vi "PDF Welding.vi"(0 "configuration file path":path caption="配置文件的路径", 1 "PDF Welding msic inf":T1) -> ()   [LabVIEW 2014]
uses:
  Ctl.xio/PDF Welding msic ctl.ctl
  SubVIS.xio/DataSocket/DataSocket_Tags.ctl
  Ctl.xio/part type.ctl
  SubVIS.xio/DataSocket/Write PLC Vars/Write Bool Var in.vi
  <vilib>/Utility/file.llb/Read From Spreadsheet File (string).vi
  SubVIS.xio/DataSocket/Write PLC Vars/Write String Var in.vi
  SubVIS.xio/DataSocket/Read PLC Vars/Read Bool Var.vi
  SubVIS.xio/DataSocket/Read PLC Vars/Read U32 Var.vi
  SubVIS.xio/DataSocket/Write PLC Vars/Write Dbl Var in.vi
  SubVIS.xio/Hopper car inf/Curing inf.vi
panel:
  in  "SQL information":string
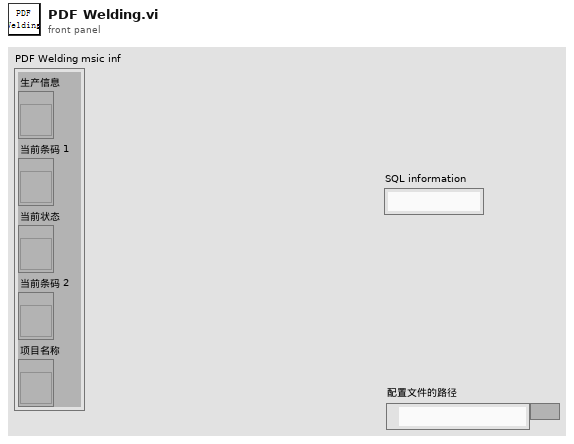
[diagram p1: front panel]
types:
  T1 = cluster{"生产信息":refnum<vi>, "当前条码 1":refnum<vi>, "当前状态":refnum<vi>, "当前条码 2":refnum<vi>, "项目名称":refnum<vi>}
  T2 = typedef "PDF Welding msic ctl.ctl" = cluster{"configuration file path":path, "DsOut":T3[], "Hopper car information":cluster{"Hopper car code":string, "Hopper car No":string, "plate No":string}, "pallet.produced number":i32, "SQL information":string, "Serial number":i32, "database path":path, "PDF Welding msic inf":cluster{"生产信息":refnum<vi>, "当前条码 1":refnum<vi>, "当前状态":refnum<vi>, "当前条码 2":refnum<vi>, "项目名称":refnum<vi>}, "Heating process parameters":cluster{"heating start":string, "heating finish":string, "Heating time use":u32}, "part type":T4, "Inlet temperature database":string[], "Outlet temperature database":string[], "Inlet temperature buffer":i32[], "Outlet temperature buffer":i32[], "PDF start time":string, "PDF finish time":string, "BarCode1":string, "BarCode2":string, "scanner resource name out":refnum<visa-resource-name>, "scanner coms or ip":string, "Outlet pressure buffer":i32[], "Outlet pressure database":string[], "scanner ip ID":refnum<k5>}
  T3 = typedef "DataSocket_Tags.ctl" = cluster{"Ds ID":refnum<k13>, "Tag":string}
  T4 = typedef "part type.ctl" = cluster{"项目号":string, "物料代码":string, "零件号":string, "供应商编码":string, "产线编码":string, "客户代码":string, "颜色代码":string, "托盘上限":i32, "加热温度":string, "加热时长":string, "EOL Stations":string}
  T5 = cluster{"Hopper car code":string, "Hopper car No":string, "plate No":string}
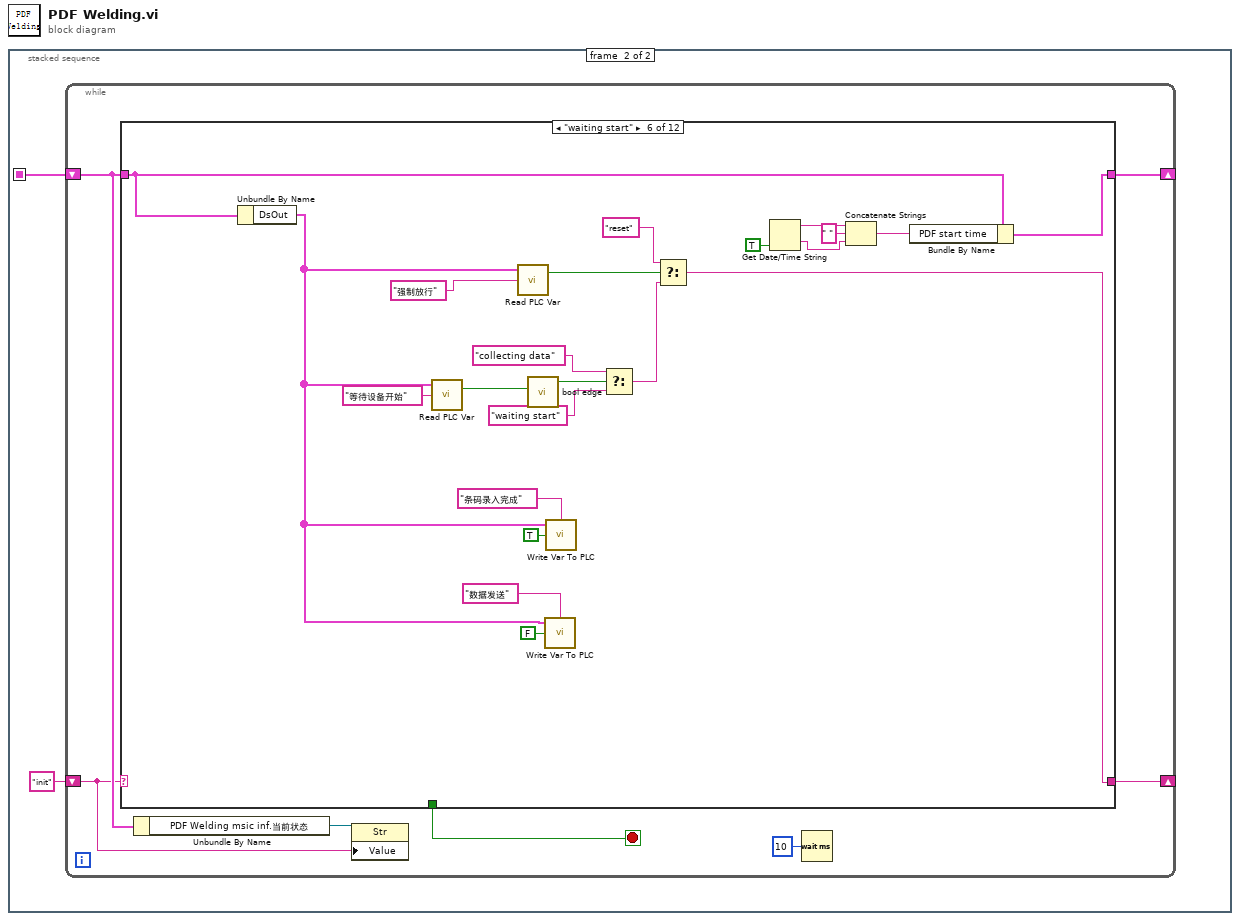
[diagram p0: block diagram]
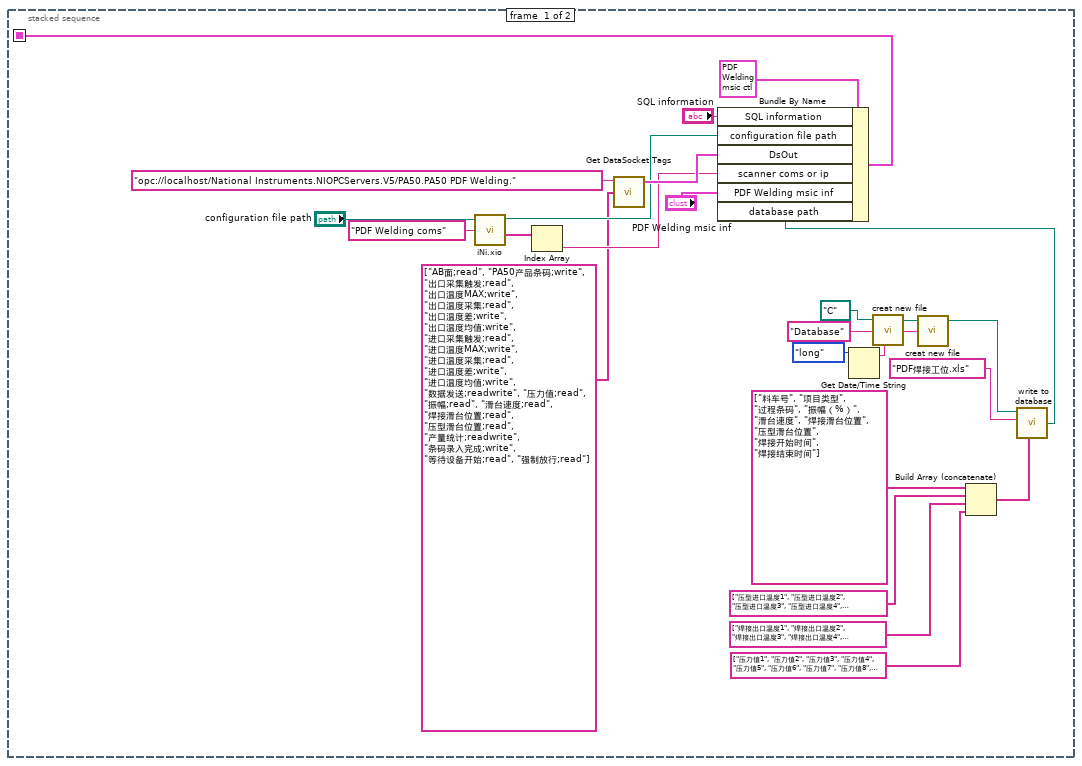
[diagram p2: hidden frame]
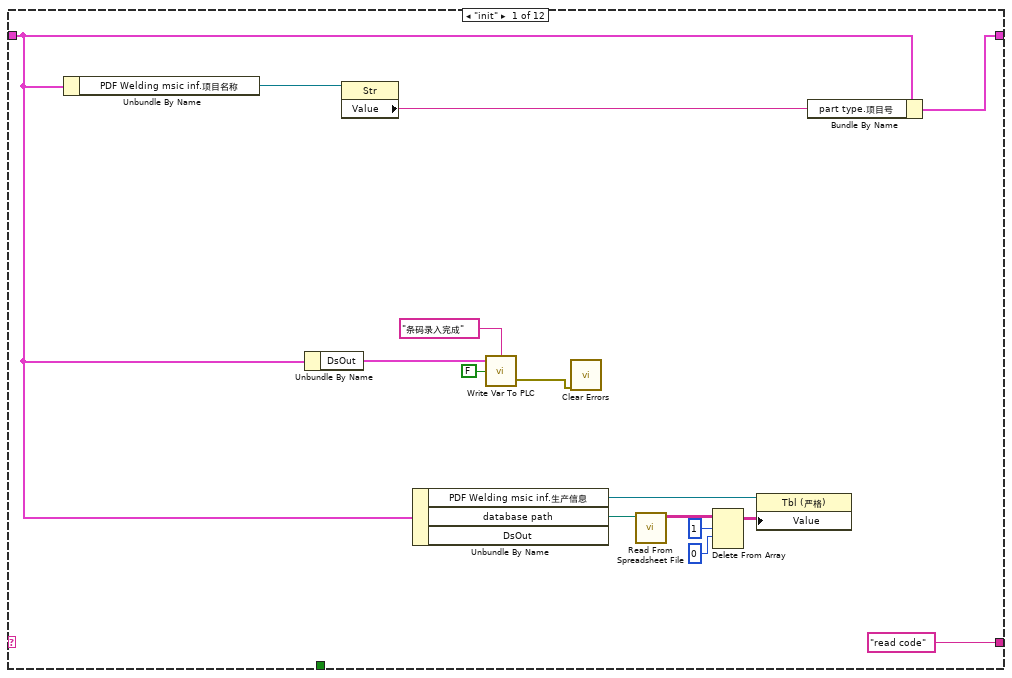
[diagram p3: hidden frame]
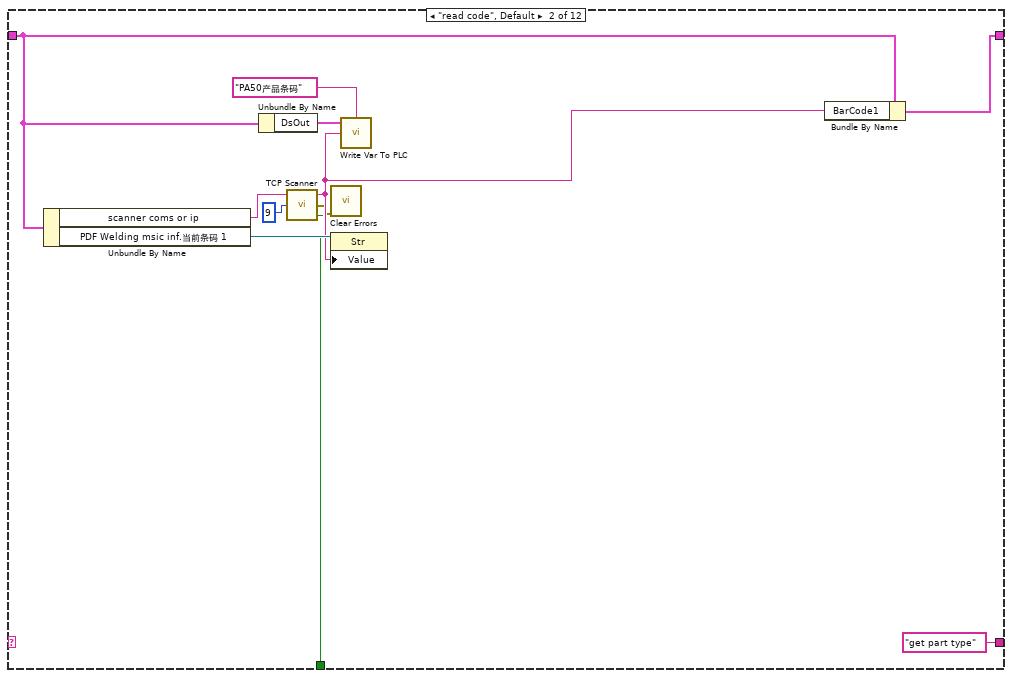
[diagram p4: hidden frame]
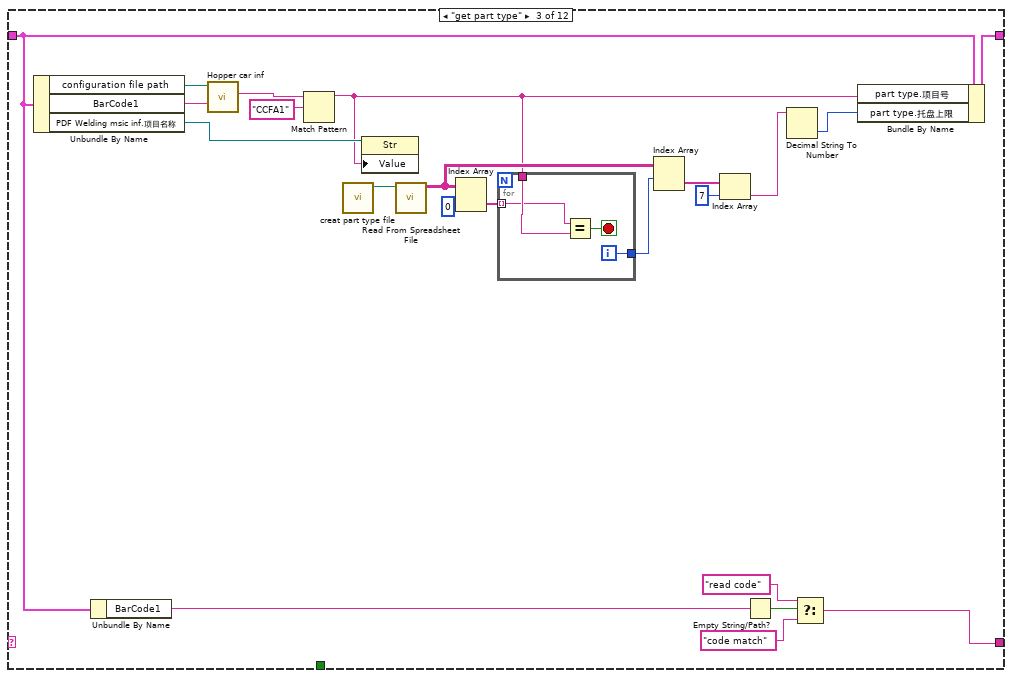
[diagram p5: hidden frame]
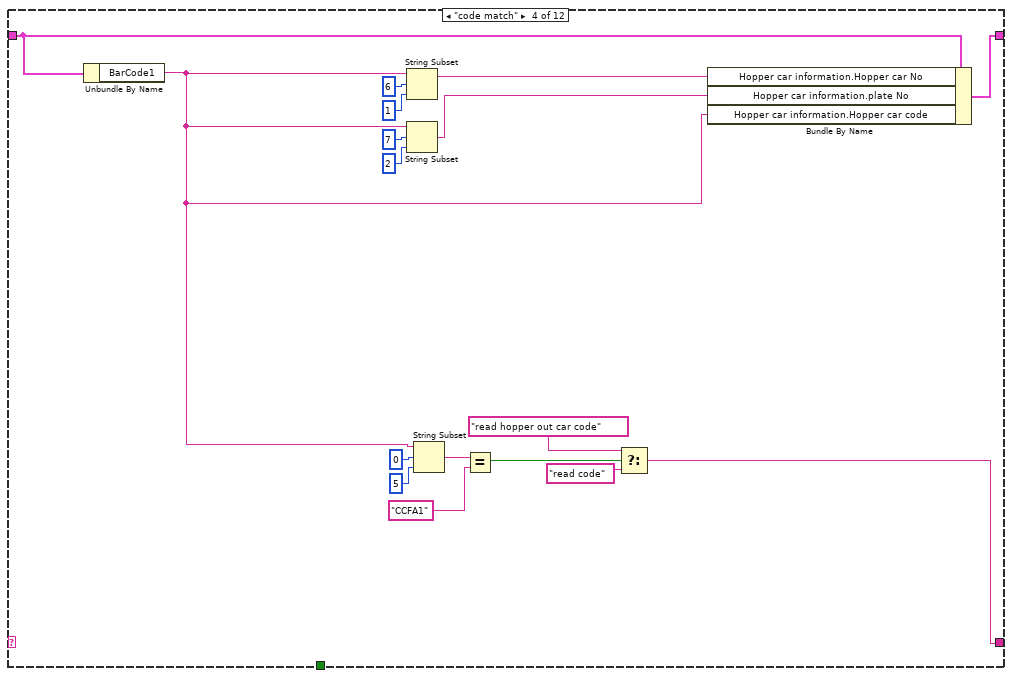
[diagram p6: hidden frame]
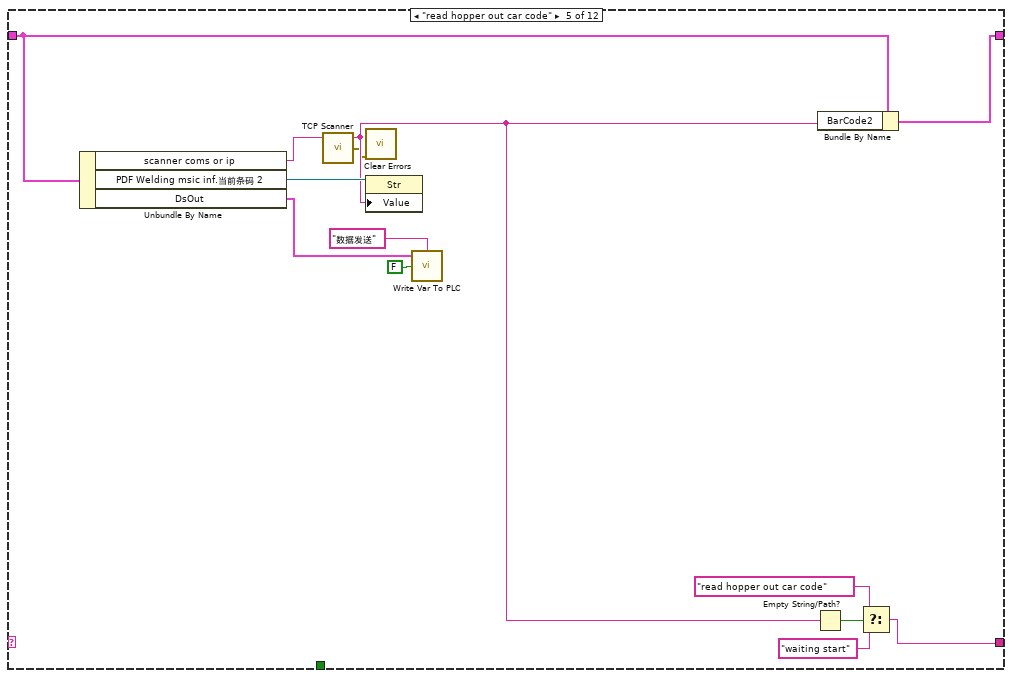
[diagram p7: hidden frame]
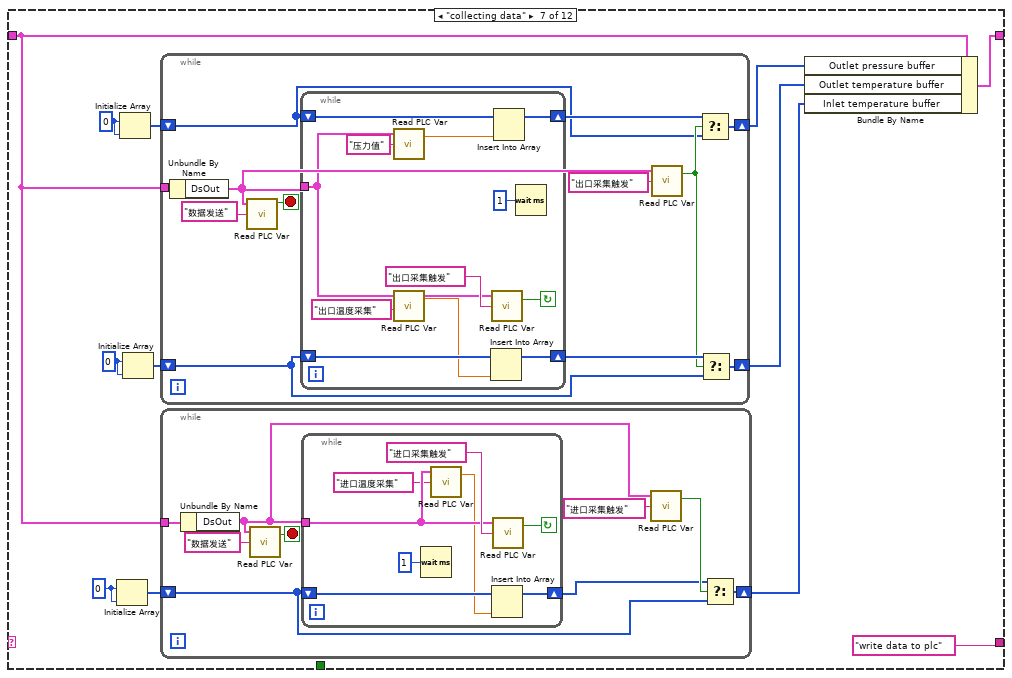
[diagram p8: hidden frame]
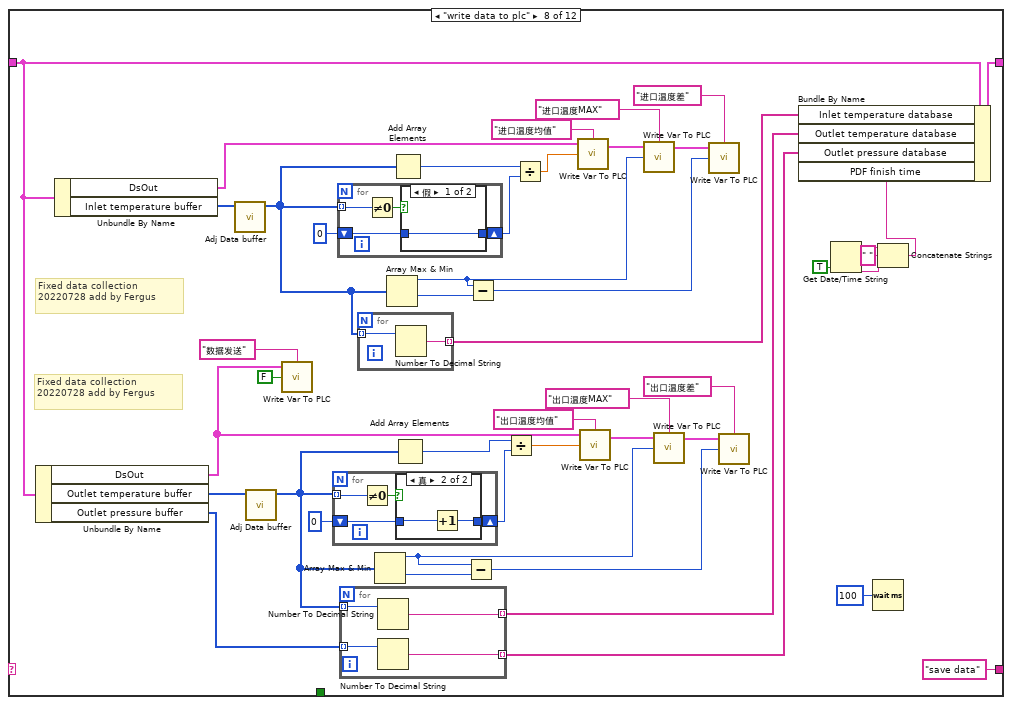
[diagram p9: hidden frame]
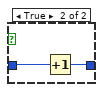
[diagram p11: hidden frame]
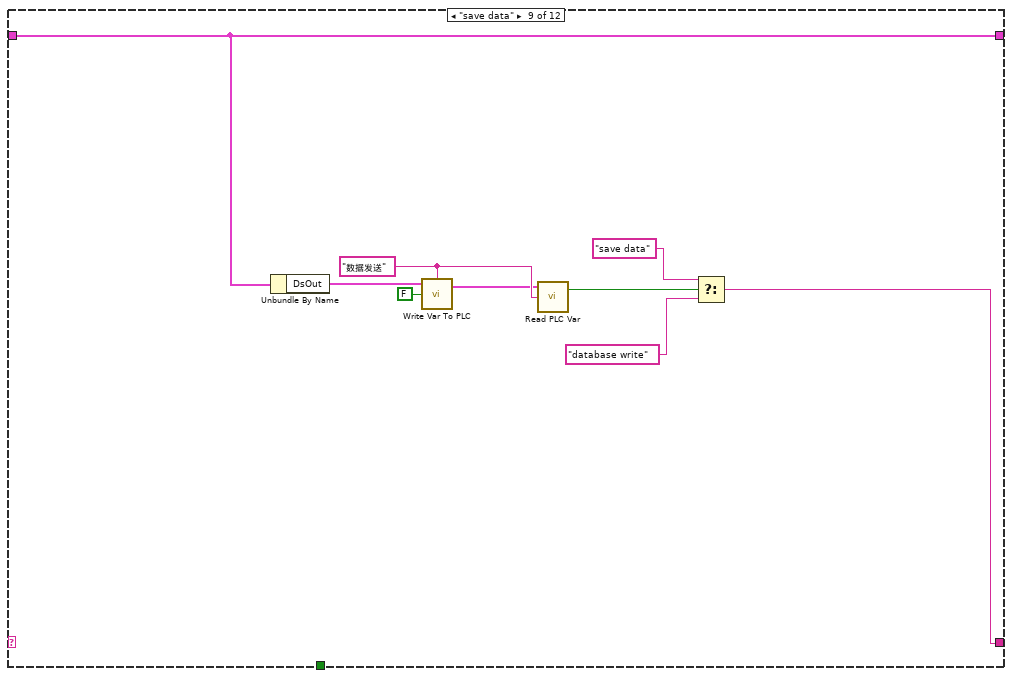
[diagram p12: hidden frame]
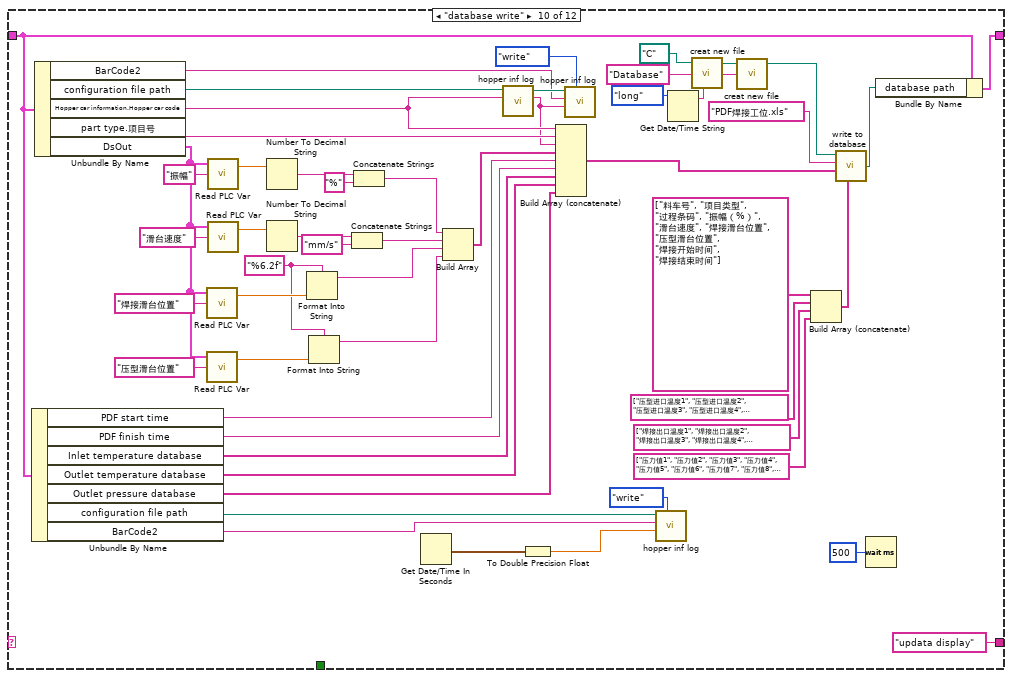
[diagram p13: hidden frame]
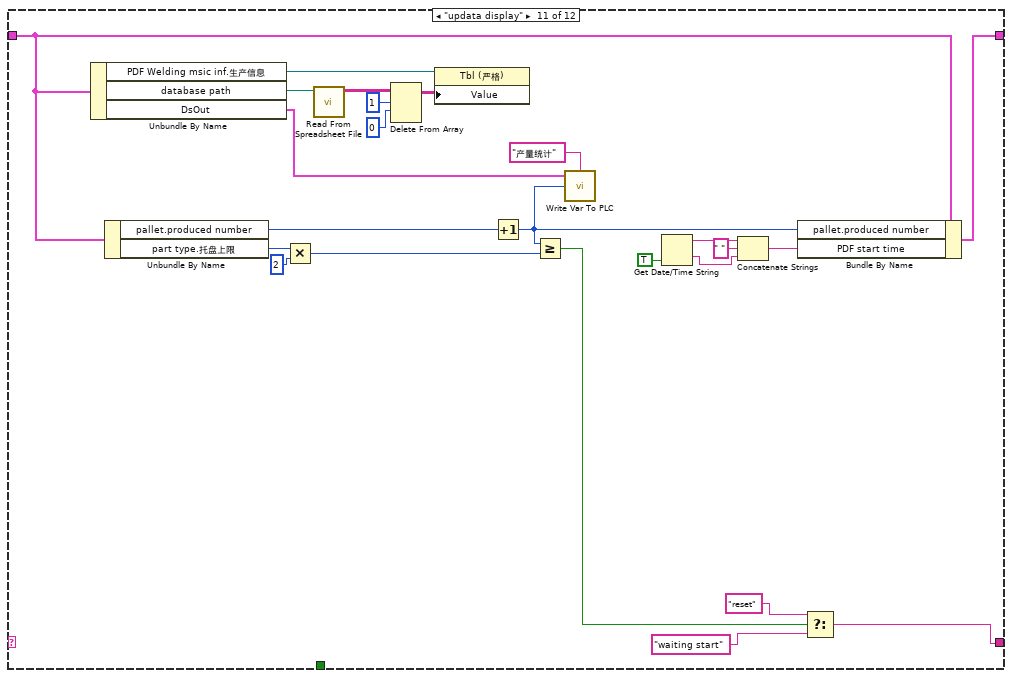
[diagram p14: hidden frame]
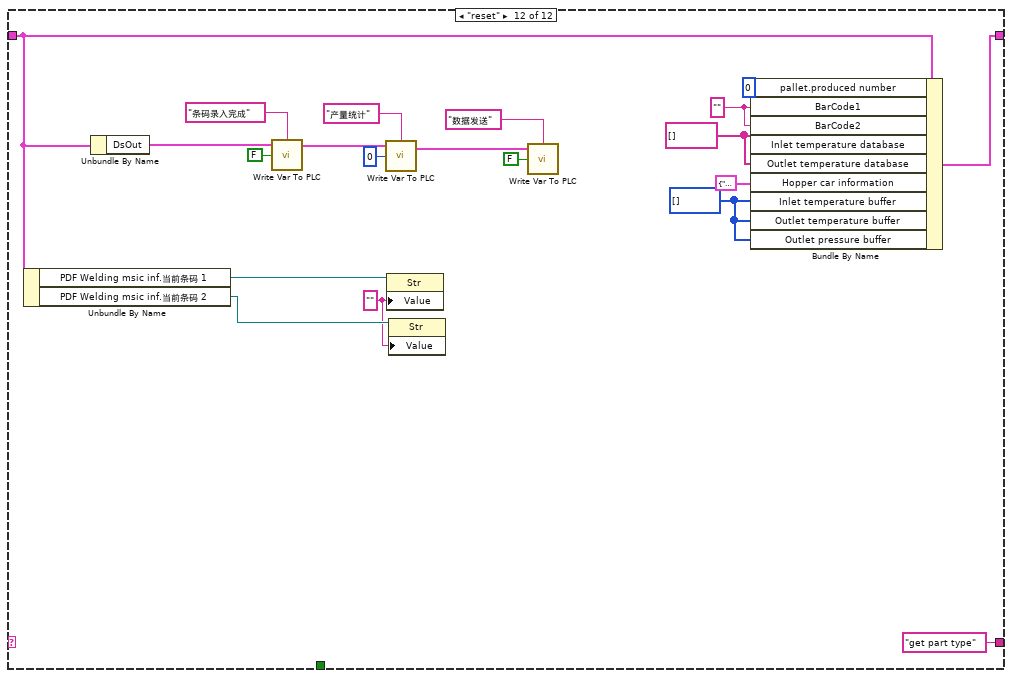
[diagram p15: hidden frame]
diagram:
  n1 = stacked-sequence {
    seq-local: [w14 _] -> [_ w26]
    frame #0 {
      n2 = call "iNi.xio.vi"("configuration file path"="configuration file path", "Sections"="PDF Welding coms") -> ("configuration file path"=w24:path, "Values"=w22:string[])  [unwired: 1 in, 3 out]
      n3 = Index Array(array=w22) -> (element=w21:string)  [unwired: 1 in]
      n4 = call "Get DataSocket Tags.vi"("All Tags"=string[] ["AB面;read", "PA50产品条码;write", "出口采集触发;read", "出口温度MAX;write", "出口温度采集;read", "出口温度差;write", "出口温度均值;write", "进口采集触发;read", "进口温度MAX;write", "进口温度采集;read", "进口温度差;write", "进口温度均值;write", "数据发送;readwrite", "压力值;read", "振幅;read", "滑台速度;read", "焊接滑台位置;read", "压型滑台位置;read", "产量统计;readwrite", "条码录入完成;write", "等待设备开始;read", "强制放行;read"], "URL"="opc://localhost/National Instruments.NIOPCServers.V5/PA50.PA50 PDF Welding.") -> ("DsOut"=w25:T3[])  [unwired: 3 in]
      n5 = Get Date/Time String(date format (0)=enum16{"short", "long", "abbreviated"}."long" ("日期格式(0)")) -> (date string=w8:string)  [unwired: 2 in, 1 out]
      n6 = call "creat new file.vi"("file name"="Database", "path"=path "C:/") -> ("created path"=w10:path)  [unwired: 1 in, 2 out]
      n7 = call "creat new file.vi"("file name"=w8, "path"=w10) -> ("created path"=w9:path)  [unwired: 1 in, 2 out]
      n8 = Build Array (concatenate)(string[] ["料车号", "项目类型", "过程条码", "振幅（%）", "滑台速度", "焊接滑台位置", "压型滑台位置", "焊接开始时间", "焊接结束时间"] ("Header"), string[] ["压型进口温度1", "压型进口温度2", "压型进口温度3", "压型进口温度4", "压型进口温度5", "压型进口温度6", "压型进口温度7", "压型进口温度8", "压型进口温度9", "压型进口温度10", "压型进口温度11", "压型进口温度12", "压型进口温度13", "压型进口温度14", "压型进口温度15", "压型进口温度16", "压型进口温度17", "压型进口温度18", "压型进口温度19", "压型进口温度20", "压型进口温度21", "压型进口温度22", "压型进口温度23", "压型进口温度24", "压型进口温度25", "压型进口温度26", "压型进口温度27", "压型进口温度28", "压型进口温度29", "压型进口温度30"] ("数组"), string[] ["焊接出口温度1", "焊接出口温度2", "焊接出口温度3", "焊接出口温度4", "焊接出口温度5", "焊接出口温度6", "焊接出口温度7", "焊接出口温度8", "焊接出口温度9", "焊接出口温度10", "焊接出口温度11", "焊接出口温度12", "焊接出口温度13", "焊接出口温度14", "焊接出口温度15", "焊接出口温度16", "焊接出口温度17", "焊接出口温度18", "焊接出口温度19", "焊接出口温度20", "焊接出口温度21", "焊接出口温度22", "焊接出口温度23", "焊接出口温度24", "焊接出口温度25", "焊接出口温度26", "焊接出口温度27", "焊接出口温度28", "焊接出口温度29", "焊接出口温度30"] ("数组"), string[] ["压力值1", "压力值2", "压力值3", "压力值4", "压力值5", "压力值6", "压力值7", "压力值8", "压力值9", "压力值10", "压力值11", "压力值12", "压力值13", "压力值14", "压力值15", "压力值16", "压力值17", "压力值18", "压力值19", "压力值20", "压力值21", "压力值22", "压力值23", "压力值24", "压力值25", "压力值26", "压力值27", "压力值28", "压力值29", "压力值30"] ("数组 2")) -> (w6:string[])
      n9 = call "write to database.vi"("Header"=w6, "file name"="PDF焊接工位.xls", "path"=w9) -> ("new file path (Not A Path if cancelled)"=w3:path)  [unwired: 3 in]
      n10 = Bundle By Name(cluster=T2 {"configuration file path"=path "", "DsOut"=[], "Hopper car information"={"Hopper car code"="", "Hopper car No"="", "plate No"=""}, "pallet.produced number"=0, "SQL information"="", "Serial number"=0, "database path"=path "", "PDF Welding msic inf"={"生产信息"=refnum, "当前条码 1"=refnum, "当前状态"=refnum, "当前条码 2"=refnum, "项目名称"=refnum}, "Heating process parameters"={"heating start"="", "heating finish"="", "Heating time use"=0}, "part type"={"项目号"="", "物料代码"="", "零件号"="", "供应商编码"="", "产线编码"="", "客户代码"="", "颜色代码"="", "托盘上限"=0, "加热温度"="", "加热时长"="", "EOL Stations"=""}, "Inlet temperature database"=[], "Outlet temperature database"=[], "Inlet temperature buffer"=[], "Outlet temperature buffer"=[], "PDF start time"="", "PDF finish time"="", "BarCode1"="", "BarCode2"="", "scanner resource name out"="", "scanner coms or ip"="", "Outlet pressure buffer"=[], "Outlet pressure database"=[], "scanner ip ID"=refnum} ("PDF Welding msic ctl"), "SQL information"="SQL information", "configuration file path"=w24, "DsOut"=w25, "scanner coms or ip"=w21, "PDF Welding msic inf"="PDF Welding msic inf", "database path"=w3) -> (w14:T2)
    }
    frame #1 {
      n11 = while {
        shift-right: [w34] -> _
        shift-left: w26 -> [w30]
        shift-right: [w33] -> _
        shift-left: "init" ("event") -> [w29]
        stop <- w28 stop-if-true
        n12 = case shown="\"waiting start\"" w29 {
          tunnel: w30 -> [w36 w57 w65 w89 w115 w119 w139 w207 w264 w308 w334 w353]
          tunnel: [w49 w60 w82 w97 w114 w117 w150 w208 w264 w314 w333 w362] -> w34
          tunnel: ["read code" "get part type" ("f") w69 w96 w108 w130 "write data to plc" ("f") "save data" ("f") w257 "updata display" ("f") w329 "get part type" ("f")] -> w33
          tunnel: [_ w50 _ _ _ _ _ _ _ _ _ _] -> w28
          frame "init" {
            n13 = Unbundle By Name(w36) -> ("PDF Welding msic inf.项目名称"=w48:refnum<vi>)
            n14 = Unbundle By Name(w36) -> ("DsOut"=w45:T3[])
            n15 = property class="Str"(reference=w48) -> ("Value"=w47:string)  [unwired: 1 in, 2 out]
            n16 = Unbundle By Name(w36) -> ("PDF Welding msic inf.生产信息"=w42:refnum<vi>, "database path"=w41:path)  [unwired: 1 out]
            n17 = call-poly "Write Var To PLC.vi"("Tag IN"="条码录入完成", "Bool Var in"=FALSE, "Ds PLCTags IN"=w45) -> ("error out"=w35:errorcluster)  [unwired: 1 in, 1 out]
            n18 = call <vilib>:"Clear Errors.vi"("error in (no error)"=w35) -> ()  [unwired: 5 in, 2 out]
            n19 = call-poly <vilib>:"Read From Spreadsheet File.vi"("file path (dialog if empty)"=w41) -> ("all rows"=w40:string[][])  [unwired: 6 in, 4 out]
            n20 = Delete From Array(array=w40, length=1 ("长度"), index (row)=0 ("索引 (行)")) -> (array with subset deleted=w37:string[][])  [unwired: 1 in, 1 out]
            n21 = property class="Tbl (严格)"(reference=w42, "Value"=w37) -> ()  [unwired: 1 in, 2 out]
            n22 = Bundle By Name(cluster=w36, "part type.项目号"=w47) -> (w49:T2)
          }
          frame "read code", Default {
            n23 = Unbundle By Name(w57) -> ("scanner coms or ip"=w53:string, "PDF Welding msic inf.当前条码 1"=w59:refnum<vi>)
            n24 = Unbundle By Name(w57) -> ("DsOut"=w56:T3[])
            n25 = call "TCP Scanner.vi"("byte of read(9)"=9 ("读取的字节"), "ip"=w53) -> ("status"=w50:bool, "错误输出"=w51:errorcluster, "Barcode"=w55:string)  [unwired: 1 in]
            n26 = call <vilib>:"Clear Errors.vi"("error in (no error)"=w51) -> ()  [unwired: 5 in, 2 out]
            n27 = property class="Str"(reference=w59, "Value"=w55) -> ()  [unwired: 1 in, 2 out]
            n28 = call-poly "Write Var To PLC.vi"("Tag IN"="PA50产品条码", "String Var in"=w55, "Ds PLCTags IN"=w56) -> ()  [unwired: 1 in, 2 out]
            n29 = Bundle By Name(cluster=w57, "BarCode1"=w55) -> (w60:T2)
          }
          frame "get part type" {
            n30 = Unbundle By Name(w65) -> ("configuration file path"=w67:path, "BarCode1"=w66:string, "PDF Welding msic inf.项目名称"=w64:refnum<vi>)
            n31 = Unbundle By Name(w65) -> ("BarCode1"=w68:string)
            n32 = call "Hopper car inf.vi"("key"=w66, "path in"=w67) -> ("value out"=w63:string)  [unwired: 8 in, 1 out]
            n33 = Match Pattern(string=w63, regular expression="CCFA1" ("正则表达式")) -> (before substring=w61:string)  [unwired: 1 in, 3 out]
            n34 = call "creat part type file.vi"() -> ("new file path (Not A Path if cancelled)"=w73:path)  [unwired: 11 in]
            n35 = property class="Str"(reference=w64, "Value"=w61) -> ()  [unwired: 1 in, 2 out]
            n36 = call-poly <vilib>:"Read From Spreadsheet File.vi"("file path (dialog if empty)"=w73) -> ("all rows"=w78:string[][])  [unwired: 6 in, 4 out]
            n37 = Index Array(array=w78, index (col)=0 ("禁用的索引 (列)")) -> (element=w80:string[])  [unwired: 1 in]
            n38 = for {
              tunnel: w80 -> [w83] mode=indexing
              tunnel: [w85] -> w77
              tunnel: w61 -> [w84]
              i -> [w85]
              stop <- w86 stop-if-true
              n39 = Equal?(x=w83, y=w84) -> (x = y?=w86:bool)
            }
            n40 = Index Array(array=w78, index (row)=w77) -> (element=w76:string[])  [unwired: 1 in]
            n41 = Index Array(array=w76, index=7 ("索引")) -> (element=w75:string)
            n42 = Empty String/Path?(string/path=w68) -> (empty?=w72:bool)
            n43 = Decimal String To Number(string=w75) -> (number=w74:i32)  [unwired: 2 in, 1 out]
            n44 = Select(t="read code", s=w72, f="code match") -> (s? t:f=w69:string)
            n45 = Bundle By Name(cluster=w65, "part type.项目号"=w61, "part type.托盘上限"=w74) -> (w82:T2)
          }
          frame "code match" {
            n46 = Unbundle By Name(w89) -> ("BarCode1"=w88:string)
            n47 = String Subset(string=w88, offset (0)=6 ("偏移量(0)"), length (rest)=1 ("长度（剩余）")) -> (substring=w91:string)
            n48 = String Subset(string=w88, offset (0)=7 ("偏移量(0)"), length (rest)=2 ("长度（剩余）")) -> (substring=w92:string)
            n49 = String Subset(string=w88, offset (0)=0 ("偏移量(0)"), length (rest)=5 ("长度（剩余）")) -> (substring=w93:string)
            n50 = Equal?(x=w93, y="CCFA1") -> (x = y?=w87:bool)
            n51 = Select(t="read hopper out car code" ("event"), s=w87, f="read code" ("event")) -> (s? t:f=w96:string)
            n52 = Bundle By Name(cluster=w89, "Hopper car information.Hopper car No"=w91, "Hopper car information.plate No"=w92, "Hopper car information.Hopper car code"=w88) -> (w97:T2)
          }
          frame "read hopper out car code" {
            n53 = Unbundle By Name(w115) -> ("scanner coms or ip"=w116:string, "PDF Welding msic inf.当前条码 2"=w113:refnum<vi>, "DsOut"=w104:T3[])
            n54 = call "TCP Scanner.vi"("ip"=w116) -> ("错误输出"=w107:errorcluster, "Barcode"=w109:string)  [unwired: 2 in, 1 out]
            n55 = call <vilib>:"Clear Errors.vi"("error in (no error)"=w107) -> ()  [unwired: 5 in, 2 out]
            n56 = property class="Str"(reference=w113, "Value"=w109) -> ()  [unwired: 1 in, 2 out]
            n57 = call-poly "Write Var To PLC.vi"("Tag IN"="数据发送", "Bool Var in"=FALSE, "Ds PLCTags IN"=w104) -> ()  [unwired: 1 in, 2 out]
            n58 = Empty String/Path?(string/path=w109) -> (empty?=w112:bool)
            n59 = Bundle By Name(cluster=w115, "BarCode2"=w109) -> (w114:T2)
            n60 = Select(t="read hopper out car code" ("f"), s=w112, f="waiting start") -> (s? t:f=w108:string)
          }
          frame "waiting start" {
            n61 = Unbundle By Name(w119) -> ("DsOut"=w124:T3[])
            n62 = call-poly "Read PLC Var.vi"("Tag IN"="等待设备开始", "Ds PLCTags IN"=w124) -> ("Bool Var out"=w137:bool)  [unwired: 1 in, 1 out]
            n63 = call-poly "Read PLC Var.vi"("Tag IN"="强制放行", "Ds PLCTags IN"=w124) -> ("Bool Var out"=w132:bool)  [unwired: 1 in, 1 out]
            n64 = call "bool edge.vi"("bool in"=w137) -> ("false-true"=w136:bool)  [unwired: 6 in, 1 out]
            n65 = call-poly "Write Var To PLC.vi"("Tag IN"="数据发送", "Bool Var in"=FALSE, "Ds PLCTags IN"=w124) -> ()  [unwired: 1 in, 2 out]
            n66 = call-poly "Write Var To PLC.vi"("Tag IN"="条码录入完成", "Bool Var in"=TRUE, "Ds PLCTags IN"=w124) -> ()  [unwired: 1 in, 2 out]
            n67 = Select(t="collecting data" ("f"), s=w136, f="waiting start") -> (s? t:f=w131:string)
            n68 = Select(t="reset" ("f"), s=w132, f=w131) -> (s? t:f=w130:string)
            n69 = Get Date/Time String(want seconds? (F)=TRUE ("需要秒？(F)")) -> (date string=w123:string, time string=w121:string)  [unwired: 2 in]
            n70 = Concatenate Strings(w123, " " ("字符串"), w121) -> (w118:string)
            n71 = Bundle By Name(cluster=w119, "PDF start time"=w118) -> (w117:T2)
          }
          frame "collecting data" {
            w142 = 0 ("维数大小")
            w144 = 0 ("维数大小")
            w147 = 0 ("维数大小")
            n72 = Initialize Array(w144, w144) -> (w143:i32[])
            n73 = Initialize Array(w142, w142) -> (w141:i32[])
            n74 = Initialize Array(w147, w147) -> (w146:i32[])
            n75 = while {
              tunnel: w139 -> [w179]
              shift-right: [w172] -> w145
              shift-left: w146 -> [w173]
              shift-right: [w171] -> w140
              shift-left: w141 -> [w168]
              stop <- w177 stop-if-true
              n76 = Unbundle By Name(w179) -> ("DsOut"=w176:T3[])
              n77 = call-poly "Read PLC Var.vi"("Tag IN"="数据发送", "Ds PLCTags IN"=w176) -> ("Bool Var out"=w177:bool)  [unwired: 1 in, 1 out]
              n78 = while {
                tunnel: w176 -> [w184]
                shift-right: [w186] -> w174
                shift-left: w173 -> [w188]
                shift-right: [w180] -> w169
                shift-left: w168 -> [w181]
                stop <- w191 continue-if-true
                n79 = call-poly "Read PLC Var.vi"("Tag IN"="压力值", "Ds PLCTags IN"=w184) -> ("U32 Var out"=w182:dbl)  [unwired: 1 in, 1 out]
                n80 = call-poly "Read PLC Var.vi"("Tag IN"="出口温度采集", "Ds PLCTags IN"=w184) -> ("U32 Var out"=w187:dbl)  [unwired: 1 in, 1 out]
                n81 = Insert Into Array(array=w188, new element=w187) -> (w186:i32[])  [unwired: 1 in]
                n82 = call-poly "Read PLC Var.vi"("Tag IN"="出口采集触发", "Ds PLCTags IN"=w184) -> ("Bool Var out"=w191:bool)  [unwired: 1 in, 1 out]
                n83 = Insert Into Array(array=w181, new element=w182) -> (w180:i32[])  [unwired: 1 in]
                n84 = Wait (ms)(milliseconds to wait=u32 1 ("等待时间（毫秒）")) -> ()  [unwired: 1 out]
              }
              n85 = call-poly "Read PLC Var.vi"("Tag IN"="出口采集触发", "Ds PLCTags IN"=w176) -> ("Bool Var out"=w170:bool)  [unwired: 1 in, 1 out]
              n86 = Select(t=w169, s=w170, f=w168) -> (s? t:f=w171:i32[])
              n87 = Select(t=w174, s=w170, f=w173) -> (s? t:f=w172:i32[])
            }
            n88 = while {
              tunnel: w139 -> [w159]
              shift-right: [w154] -> w149
              shift-left: w143 -> [w151]
              stop <- w157 stop-if-true
              n89 = Unbundle By Name(w159) -> ("DsOut"=w156:T3[])
              n90 = call-poly "Read PLC Var.vi"("Tag IN"="数据发送", "Ds PLCTags IN"=w156) -> ("Bool Var out"=w157:bool)  [unwired: 1 in, 1 out]
              n91 = while {
                tunnel: w156 -> [w165]
                shift-right: [w161] -> w152
                shift-left: w151 -> [w163]
                stop <- w167 continue-if-true
                n92 = Wait (ms)(milliseconds to wait=u32 1 ("等待时间（毫秒）")) -> ()  [unwired: 1 out]
                n93 = call-poly "Read PLC Var.vi"("Tag IN"="进口温度采集", "Ds PLCTags IN"=w165) -> ("U32 Var out"=w162:dbl)  [unwired: 1 in, 1 out]
                n94 = Insert Into Array(array=w163, new element=w162) -> (w161:i32[])  [unwired: 1 in]
                n95 = call-poly "Read PLC Var.vi"("Tag IN"="进口采集触发", "Ds PLCTags IN"=w165) -> ("Bool Var out"=w167:bool)  [unwired: 1 in, 1 out]
              }
              n96 = call-poly "Read PLC Var.vi"("Tag IN"="进口采集触发", "Ds PLCTags IN"=w156) -> ("Bool Var out"=w153:bool)  [unwired: 1 in, 1 out]
              n97 = Select(t=w152, s=w153, f=w151) -> (s? t:f=w154:i32[])
            }
            n98 = Bundle By Name(cluster=w139, "Outlet pressure buffer"=w140, "Outlet temperature buffer"=w145, "Inlet temperature buffer"=w149) -> (w150:T2)
          }
          frame "write data to plc" {
            # "Fixed data collection\n20220728 add by Fergus"
            # "Fixed data collection\n20220728 add by Fergus"
            n99 = Unbundle By Name(w207) -> ("DsOut"=w204:T3[], "Outlet temperature buffer"=w193:i32[], "Outlet pressure buffer"=w198:i32[])
            n100 = Unbundle By Name(w207) -> ("DsOut"=w232:T3[], "Inlet temperature buffer"=w195:i32[])
            n101 = call "Adj Data buffer.vi"("data buffer"=w195) -> ("data buffer out"=w194:i32[])  [unwired: 10 in]
            n102 = call "Adj Data buffer.vi"("data buffer"=w193) -> ("data buffer out"=w192:i32[])  [unwired: 10 in]
            n103 = call-poly "Write Var To PLC.vi"("Tag IN"="数据发送", "Bool Var in"=FALSE, "Ds PLCTags IN"=w204) -> ()  [unwired: 1 in, 2 out]
            n104 = for {
              tunnel: w192 -> [w246] mode=indexing
              shift-right: [w243] -> w227
              shift-left: 0 -> [w244]
              n105 = Not Equal To 0?(x=w246) -> (x != 0?=w245:bool)
              n106 = case shown="真" w245 {
                tunnel: w244 -> [w247 w248]
                tunnel: [w247 w249] -> w243
                frame False {
                }
                frame True {
                  n107 = Increment(x=w248) -> (x+1=w249:i32)
                }
              }
            }
            n108 = for {
              tunnel: w194 -> [w253] mode=indexing
              shift-right: [w250] -> w234
              shift-left: 0 -> [w251]
              n109 = Not Equal To 0?(x=w253) -> (x != 0?=w252:bool)
              n110 = case shown="假" w252 {
                tunnel: w251 -> [w254 w255]
                tunnel: [w254 w256] -> w250
                frame False {
                }
                frame True {
                  n111 = Increment(x=w255) -> (x+1=w256:i32)
                }
              }
            }
            n112 = for {
              tunnel: w192 -> [w240] mode=indexing
              tunnel: [w238] -> w210 mode=indexing
              tunnel: w198 -> [w239] mode=indexing
              tunnel: [w237] -> w196 mode=indexing
              n113 = Number To Decimal String(number=w240) -> (decimal integer string=w238:string)  [unwired: 1 in]
              n114 = Number To Decimal String(number=w239) -> (decimal integer string=w237:string)  [unwired: 1 in]
            }
            n115 = for {
              tunnel: w194 -> [w242] mode=indexing
              tunnel: [w241] -> w211 mode=indexing
              n116 = Number To Decimal String(number=w242) -> (decimal integer string=w241:string)  [unwired: 1 in]
            }
            n117 = Array Max & Min(array=w192) -> (max value=w214:i32, min value=w213:i32)  [unwired: 2 out]
            n118 = Array Max & Min(array=w194) -> (max value=w222:i32, min value=w225:i32)  [unwired: 2 out]
            n119 = Add Array Elements(numeric array=w194) -> (sum=w233:i32)
            n120 = Add Array Elements(numeric array=w192) -> (sum=w228:i32)
            n121 = Subtract(x=w214, y=w213) -> (x-y=w212:i32)
            n122 = Subtract(x=w222, y=w225) -> (x-y=w219:i32)
            n123 = Divide(x=w228, y=w227) -> (x/y=w226:dbl)
            n124 = Divide(x=w233, y=w234) -> (x/y=w230:dbl)
            n125 = call-poly "Write Var To PLC.vi"("Tag IN"="进口温度均值", "Dbl Var in"=w230, "Ds PLCTags IN"=w232) -> ("Ds PLCTags OUT"=w224:T3[])  [unwired: 1 in, 1 out]
            n126 = call-poly "Write Var To PLC.vi"("Tag IN"="出口温度均值", "Dbl Var in"=w226, "Ds PLCTags IN"=w204) -> ("Ds PLCTags OUT"=w215:T3[])  [unwired: 1 in, 1 out]
            n127 = call-poly "Write Var To PLC.vi"("Tag IN"="进口温度MAX", "Dbl Var in"=w222, "Ds PLCTags IN"=w224) -> ("Ds PLCTags OUT"=w221:T3[])  [unwired: 1 in, 1 out]
            n128 = call-poly "Write Var To PLC.vi"("Tag IN"="出口温度MAX", "Dbl Var in"=w214, "Ds PLCTags IN"=w215) -> ("Ds PLCTags OUT"=w217:T3[])  [unwired: 1 in, 1 out]
            n129 = call-poly "Write Var To PLC.vi"("Tag IN"="进口温度差", "Dbl Var in"=w219, "Ds PLCTags IN"=w221) -> ()  [unwired: 1 in, 2 out]
            n130 = call-poly "Write Var To PLC.vi"("Tag IN"="出口温度差", "Dbl Var in"=w212, "Ds PLCTags IN"=w217) -> ()  [unwired: 1 in, 2 out]
            n131 = Get Date/Time String(want seconds? (F)=TRUE ("需要秒？(F)")) -> (date string=w203:string, time string=w201:string)  [unwired: 2 in]
            n132 = Wait (ms)(milliseconds to wait=u32 100 ("等待时间（毫秒）")) -> ()  [unwired: 1 out]
            n133 = Concatenate Strings(w203, " " ("字符串"), w201) -> (w199:string)
            n134 = Bundle By Name(cluster=w207, "Inlet temperature database"=w211, "Outlet temperature database"=w210, "Outlet pressure database"=w196, "PDF finish time"=w199) -> (w208:T2)
          }
          frame "save data" {
            w262 = "数据发送" ("Tag IN")
            n135 = Unbundle By Name(w264) -> ("DsOut"=w263:T3[])
            n136 = call-poly "Write Var To PLC.vi"("Tag IN"=w262, "Bool Var in"=FALSE, "Ds PLCTags IN"=w263) -> ("Ds PLCTags OUT"=w261:T3[])  [unwired: 1 in, 1 out]
            n137 = call-poly "Read PLC Var.vi"("Tag IN"=w262, "Ds PLCTags IN"=w261) -> ("Bool Var out"=w260:bool)  [unwired: 1 in, 1 out]
            n138 = Select(t="save data" ("f"), s=w260, f="database write") -> (s? t:f=w257:string)
          }
          frame "database write" {
            w271 = "%6.2f" ("格式字符串")
            n139 = Unbundle By Name(w308) -> ("PDF start time"=w304:string, "PDF finish time"=w303:string, "Inlet temperature database"=w302:string[], "Outlet temperature database"=w301:string[], "Outlet pressure database"=w268:string[], "configuration file path"=w289:path, "BarCode2"=w286:string)
            n140 = Unbundle By Name(w308) -> ("BarCode2"=w296:string, "configuration file path"=w307:path, "Hopper car information.Hopper car code"=w306:string, "part type.项目号"=w305:string, "DsOut"=w295:T3[])
            n141 = call-poly "Read PLC Var.vi"("Tag IN"="焊接滑台位置", "Ds PLCTags IN"=w295) -> ("U32 Var out"=w274:dbl)  [unwired: 1 in, 1 out]
            n142 = call-poly "Read PLC Var.vi"("Tag IN"="压型滑台位置", "Ds PLCTags IN"=w295) -> ("U32 Var out"=w272:dbl)  [unwired: 1 in, 1 out]
            n143 = call-poly "Read PLC Var.vi"("Tag IN"="振幅", "Ds PLCTags IN"=w295) -> ("U32 Var out"=w283:dbl)  [unwired: 1 in, 1 out]
            n144 = call-poly "Read PLC Var.vi"("Tag IN"="滑台速度", "Ds PLCTags IN"=w295) -> ("U32 Var out"=w280:dbl)  [unwired: 1 in, 1 out]
            n145 = Number To Decimal String(number=w283) -> (decimal integer string=w282:string)  [unwired: 1 in]
            n146 = Number To Decimal String(number=w280) -> (decimal integer string=w279:string)  [unwired: 1 in]
            n147 = Format Into String(format string=w271, w274) -> (resulting string=w273:string)  [unwired: 2 in, 1 out]
            n148 = Format Into String(format string=w271, w272) -> (resulting string=w270:string)  [unwired: 2 in, 1 out]
            n149 = Concatenate Strings(w279, "mm/s" ("字符串")) -> (w276:string)
            n150 = Concatenate Strings(w282, "%" ("字符串")) -> (w277:string)
            n151 = Get Date/Time In Seconds() -> (seconds since 1Jan1904=w288:timestamp)
            n152 = Build Array(w277, w276, w273, w270) -> (w275:string[])
            n153 = call-poly "hopper inf log.vi"("key"=w306, "path in"=w307) -> ("value out"=w290:string, "path out"=w298:path)  [unwired: 8 in]
            n154 = To Double Precision Float(number=w288) -> (double precision float=w287:dbl)
            n155 = Build Array (concatenate)(w306, w305, w290, w275, w304, w303, w302, w301, w268) -> (w300:string[])
            n156 = call-poly "hopper inf log.vi"("write\\read（read)"=enum16{"read", "write"}."write" ("write\\read（read)"), "value"=w290, "key"=w296, "path in"=w298) -> ()  [unwired: 6 in, 2 out]
            n157 = call-poly "hopper inf log.vi"("write\\read（read)"=enum16{"read", "write"}."write" ("write\\read（read)"), "value in"=w287, "key"=w286, "path in"=w289) -> ()  [unwired: 6 in, 2 out]
            n158 = Get Date/Time String(date format (0)=enum16{"short", "long", "abbreviated"}."long" ("日期格式(0)")) -> (date string=w311:string)  [unwired: 2 in, 1 out]
            n159 = call "creat new file.vi"("file name"="Database", "path"=path "C:/") -> ("created path"=w313:path)  [unwired: 1 in, 2 out]
            n160 = call "creat new file.vi"("file name"=w311, "path"=w313) -> ("created path"=w312:path)  [unwired: 1 in, 2 out]
            n161 = Build Array (concatenate)(string[] ["料车号", "项目类型", "过程条码", "振幅（%）", "滑台速度", "焊接滑台位置", "压型滑台位置", "焊接开始时间", "焊接结束时间"] ("Header"), string[] ["压型进口温度1", "压型进口温度2", "压型进口温度3", "压型进口温度4", "压型进口温度5", "压型进口温度6", "压型进口温度7", "压型进口温度8", "压型进口温度9", "压型进口温度10", "压型进口温度11", "压型进口温度12", "压型进口温度13", "压型进口温度14", "压型进口温度15", "压型进口温度16", "压型进口温度17", "压型进口温度18", "压型进口温度19", "压型进口温度20", "压型进口温度21", "压型进口温度22", "压型进口温度23", "压型进口温度24", "压型进口温度25", "压型进口温度26", "压型进口温度27", "压型进口温度28", "压型进口温度29", "压型进口温度30"] ("数组"), string[] ["焊接出口温度1", "焊接出口温度2", "焊接出口温度3", "焊接出口温度4", "焊接出口温度5", "焊接出口温度6", "焊接出口温度7", "焊接出口温度8", "焊接出口温度9", "焊接出口温度10", "焊接出口温度11", "焊接出口温度12", "焊接出口温度13", "焊接出口温度14", "焊接出口温度15", "焊接出口温度16", "焊接出口温度17", "焊接出口温度18", "焊接出口温度19", "焊接出口温度20", "焊接出口温度21", "焊接出口温度22", "焊接出口温度23", "焊接出口温度24", "焊接出口温度25", "焊接出口温度26", "焊接出口温度27", "焊接出口温度28", "焊接出口温度29", "焊接出口温度30"] ("数组"), string[] ["压力值1", "压力值2", "压力值3", "压力值4", "压力值5", "压力值6", "压力值7", "压力值8", "压力值9", "压力值10", "压力值11", "压力值12", "压力值13", "压力值14", "压力值15", "压力值16", "压力值17", "压力值18", "压力值19", "压力值20", "压力值21", "压力值22", "压力值23", "压力值24", "压力值25", "压力值26", "压力值27", "压力值28", "压力值29", "压力值30"] ("数组 2")) -> (w309:string[])
            n162 = call "write to database.vi"("Header"=w309, "data in"=w300, "file name"="PDF焊接工位.xls", "path"=w312) -> ("new file path (Not A Path if cancelled)"=w315:path)  [unwired: 2 in]
            n163 = Wait (ms)(milliseconds to wait=u32 500 ("等待时间（毫秒）")) -> ()  [unwired: 1 out]
            n164 = Bundle By Name(cluster=w308, "database path"=w315) -> (w314:T2)
          }
          frame "updata display" {
            n165 = Unbundle By Name(w334) -> ("PDF Welding msic inf.生产信息"=w343:refnum<vi>, "database path"=w342:path, "DsOut"=w327:T3[])
            n166 = Unbundle By Name(w334) -> ("pallet.produced number"=w328:i32, "part type.托盘上限"=w337:i32)
            n167 = Multiply(x=w337, y=2) -> (x*y=w335:i32)
            n168 = call-poly <vilib>:"Read From Spreadsheet File.vi"("file path (dialog if empty)"=w342) -> ("all rows"=w341:string[][])  [unwired: 6 in, 4 out]
            n169 = Delete From Array(array=w341, length=1 ("长度"), index (row)=0 ("索引 (行)")) -> (array with subset deleted=w338:string[][])  [unwired: 1 in, 1 out]
            n170 = property class="Tbl (严格)"(reference=w343, "Value"=w338) -> ()  [unwired: 1 in, 2 out]
            n171 = Increment(x=w328) -> (x+1=w325:i32)
            n172 = Greater Or Equal?(x=w325, y=w335) -> (x >= y?=w332:bool)
            n173 = call-poly "Write Var To PLC.vi"("Tag IN"="产量统计", "Dbl Var in"=w325, "Ds PLCTags IN"=w327) -> ()  [unwired: 1 in, 2 out]
            n174 = Get Date/Time String(want seconds? (F)=TRUE ("需要秒？(F)")) -> (date string=w324:string, time string=w322:string)  [unwired: 2 in]
            n175 = Concatenate Strings(w324, " " ("字符串"), w322) -> (w320:string)
            n176 = Bundle By Name(cluster=w334, "pallet.produced number"=w325, "PDF start time"=w320) -> (w333:T2)
            n177 = Select(t="reset" ("f"), s=w332, f="waiting start") -> (s? t:f=w329:string)
          }
          frame "reset" {
            w350 = "" ("值")
            w357 = i32[] [] ("Inlet temperature buffer")
            w359 = string[] [] ("Database")
            w358 = "" ("BarCode")
            n178 = Unbundle By Name(w353) -> ("PDF Welding msic inf.当前条码 1"=w352:refnum<vi>, "PDF Welding msic inf.当前条码 2"=w351:refnum<vi>)
            n179 = Unbundle By Name(w353) -> ("DsOut"=w356:T3[])
            n180 = call-poly "Write Var To PLC.vi"("Tag IN"="条码录入完成", "Bool Var in"=FALSE, "Ds PLCTags IN"=w356) -> ("Ds PLCTags OUT"=w349:T3[])  [unwired: 1 in, 1 out]
            n181 = call-poly "Write Var To PLC.vi"("Tag IN"="产量统计", "Dbl Var in"=0, "Ds PLCTags IN"=w349) -> ("Ds PLCTags OUT"=w344:T3[])  [unwired: 1 in, 1 out]
            n182 = property class="Str"(reference=w352, "Value"=w350) -> ()  [unwired: 1 in, 2 out]
            n183 = property class="Str"(reference=w351, "Value"=w350) -> ()  [unwired: 1 in, 2 out]
            n184 = call-poly "Write Var To PLC.vi"("Tag IN"="数据发送", "Bool Var in"=FALSE, "Ds PLCTags IN"=w344) -> ()  [unwired: 1 in, 2 out]
            n185 = Bundle By Name(cluster=w353, "pallet.produced number"=0, "BarCode1"=w358, "BarCode2"=w358, "Inlet temperature database"=w359, "Outlet temperature database"=w359, "Hopper car information"=T5 {"Hopper car code"="", "Hopper car No"="", "plate No"=""}, "Inlet temperature buffer"=w357, "Outlet temperature buffer"=w357, "Outlet pressure buffer"=w357) -> (w362:T2)
          }
        }
        n186 = Unbundle By Name(w30) -> ("PDF Welding msic inf.当前状态"=w31:refnum<vi>)
        n187 = property class="Str"(reference=w31, "Value"=w29) -> ()  [unwired: 1 in, 2 out]
        n188 = Wait (ms)(milliseconds to wait=u32 10 ("等待时间（毫秒）")) -> ()  [unwired: 1 out]
      }
    }
  }
